vi "CleanUp.vi"(8 "error in (no error)":errorcluster, 11 "TestCase in":refnum<class "TestCase.lvclass">) -> (0 "error out":errorcluster, 3 "TestCase out":refnum<class "TestCase.lvclass">)   [LabVIEW 2013, in "TestCase.lvclass"]
uses:
  TestCase.lvclass
  TestCase.lvclass/TestCase.ctl
panel:
  # "JKI VI Tester for LabVIEW\nhttp://jkisoft.com/vi-tester\nCopyright (C) 2007-2009, JKI <info@jkisoft.com>\nALL RIGHTS RESERVED"
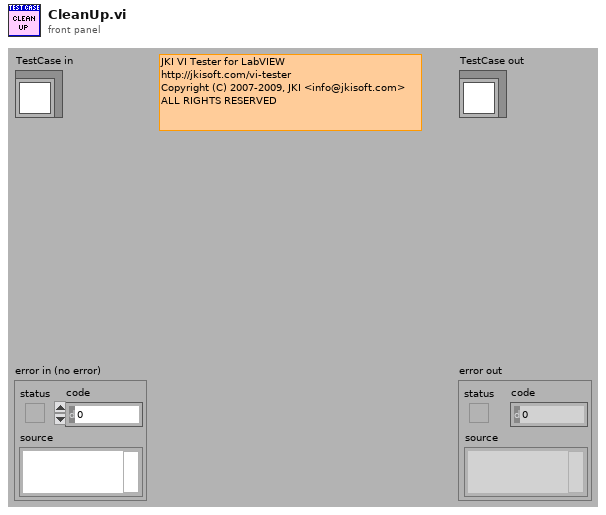
[diagram p1: front panel]
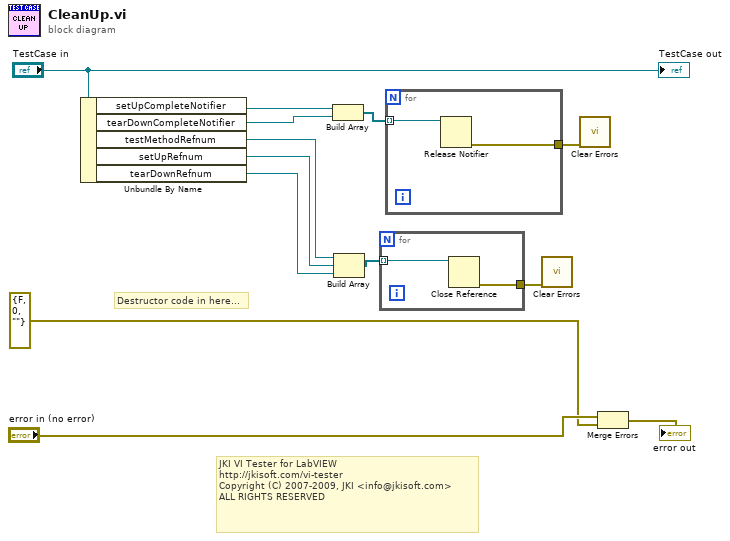
[diagram p0: block diagram]
diagram:
  # "JKI VI Tester for LabVIEW\nhttp://jkisoft.com/vi-tester\nCopyright (C) 2007-2009, JKI <info@jkisoft.com>\nALL RIGHTS RESERVED"
  # "Destructor code in here..."
  n1 = Unbundle By Name("TestCase in") -> ("setUpCompleteNotifier"=w9:refnum<notifier>, "tearDownCompleteNotifier"=w8:refnum<notifier>, "testMethodRefnum"=w5:refnum<vi>, "setUpRefnum"=w4:refnum<vi>, "tearDownRefnum"=w3:refnum<vi>)
  n2 = Build Array(w9, w8) -> (w7:refnum<notifier>[])
  n3 = Build Array(w5, w4, w3) -> (w2:refnum<vi>[])
  n4 = for {
    tunnel: w2 -> [w15] mode=indexing
    tunnel: [w14] -> w1
    n5 = Close Reference(reference=w15) -> (error out=w14:errorcluster)  [unwired: 1 in]
  }
  n6 = for {
    tunnel: w7 -> [w17] mode=indexing
    tunnel: [w16] -> w6
    n7 = Release Notifier(notifier=w17) -> (error out=w16:errorcluster)  [unwired: 2 in, 2 out]
  }
  n8 = call <vilib>:"Clear Errors.vi"("error in (no error)"=w1) -> ()  [unwired: 6 in, 1 out]
  n9 = call <vilib>:"Clear Errors.vi"("error in (no error)"=w6) -> ()  [unwired: 6 in, 1 out]
  n10 = Merge Errors("error in (no error)", errorcluster {"status"=FALSE, "code"=0, "source"=""} ("error in (no error)")) -> (→"error out":errorcluster)
  "TestCase out" <- "TestCase in"
